vi "Read Routed Trigger.vi"(0 "immediate trigger":bool, 1 "trigger source type":T1, 5 "software trigger":bool, 7 "digital trigger":bool, 9 "data trigger":bool, 12 "digital trigger on rising edge":bool, 13 "digital trigger on level high":bool) -> (4 "trigger":bool)   [LabVIEW 2023, in "niUSRP Rx Core v1 FPGA.lvclass"]
doc: "this VI selects the host-requested trigger.\n\n<b>trigger source type:</b> dictates which trigger source to use. this signal should be connected to a host-controlled register/control.\n\n<b>digital edge trigger on rising edge:</b> the polarity of the digital edge trigger.\n\n<b>digital trigger on level high:</b> the level of digital level trigger. trigger asserts accordingly.\n\n<b>digital trigger:</b> this signal is conditioned such that a pulse is generated for Edge and a level is held for Level. if 'trigger source type' is configured to Digital Level then trigger will assert when the 'digital trigger on level high' criterion is met. this signal is typically generated inside the FPGA. if 'trigger source type' is configured to Digital Edge then trigger will assert when polarity criterion is met as configured by 'digital trigger on rising edge'. this signal typically comes from an IO port or Routing.\n\n<b>software trigger:</b> circuitry places a rising edge detect on the incoming signal. <b>this trigger will override all other trigger sources.</b>\n\n<b>immediate trigger source:</b> circuitry places a rising edge detect on the incoming signal. this signal is typically driven by a 'ready for' signal from a Data Engine.\n\n<b>data trigger:</b> this can be used in a variety of ways, there is no edge detection on this signal."
uses:
  <instrlib>/niUSRP/Reference FPGA/Rx Core/niUSRP Rx Core v1 FPGA.lvclass
  <instrlib>/niVST/Reference FPGA/FPGA/niUSRP Rx Core v1 FPGA/Public/Typedefs/Trigger Source Type.ctl
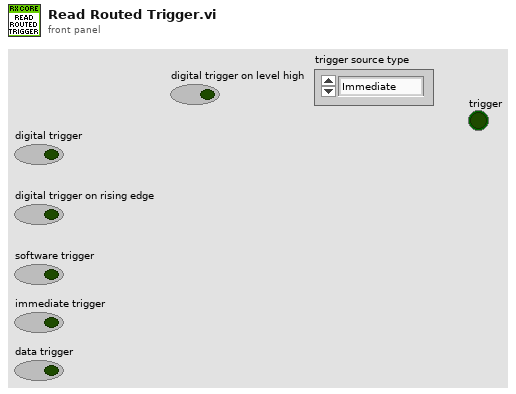
[diagram p1: front panel]
types:
  T1 = typedef "niUSRP Rx Core v1 FPGA.lvclass/Trigger Source Type.ctl" = enum8{"Immediate", "Software", "Digital Edge", "IQ Power Edge", "Digital Level", "IQ Analog Edge", "Custom"}
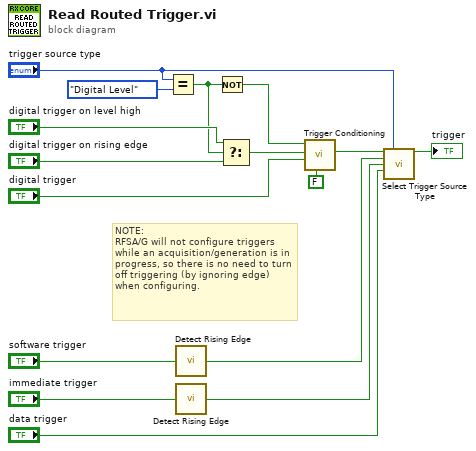
[diagram p0: block diagram]
diagram:
  # "NOTE:\nRFSA/G will not configure triggers while an acquisition/generation is in progress, so there is no need to turn off triggering (by ignoring edge) when configuring."
  n1 = Equal?(x="trigger source type", y=Trigger_Source_Type."Digital Level" ("trigger source type")) -> (x = y?=w1:bool)
  n2 = call <instrlib>:"Detect Rising Edge.vi"("signal"="software trigger") -> ("edge detected"=w11:bool)  [unwired: 14 in]
  n3 = call <instrlib>:"Detect Rising Edge.vi"("signal"="immediate trigger") -> ("edge detected"=w9:bool)  [unwired: 14 in]
  n4 = Not(x=w1) -> (.not. x?=w2:bool)
  n5 = Select(t="digital trigger on level high", s=w1, f="digital trigger on rising edge") -> (s? t:f=w3:bool)
  n6 = call <instrlib>:"Trigger Conditioning.vi"("ignore edge"=FALSE, "signal in"="digital trigger", "polarity"=w3, "edge sensitive?"=w2) -> ("signal out"=w13:bool)  [unwired: 7 in]
  n7 = call <instrlib>:"Select Trigger Source Type.vi"("digital trigger source"=w13, "trigger source type"="trigger source type", "software trigger source"=w11, "immediate trigger source"=w9, "data trigger source"="data trigger") -> ("trigger"=→"trigger":bool)  [unwired: 10 in]
